vi "create systems from points.vi"(1 "points":cluster{"x":dbl, "f(x)":dbl}[](array[cluster])) -> (0 "systems of equations":T1[](array[typedef]))   [LabVIEW 2009]
uses:
  polynomial equation.ctl
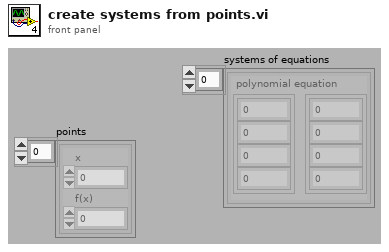
[diagram p1: front panel]
types:
  T1 = typedef "polynomial equation.ctl" = cluster{"i":dbl[], "ii":dbl[]}
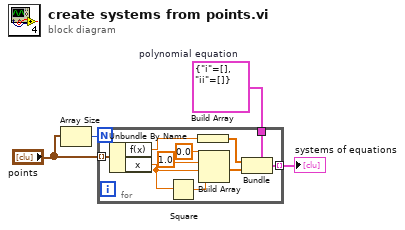
[diagram p0: block diagram]
diagram:
  w3 = T1 {"i"=[], "ii"=[]}  # polynomial equation
  n1 = Array Size(array="points") -> (size(s)=w2:i32)
  n2 = for {
    N: w2 -> [_]
    tunnel: "points" -> [w14] mode=indexing
    tunnel: w3 -> [w9]
    tunnel: [w6] -> w4 mode=indexing
    n3 = Unbundle By Name(w14) -> ("f(x)"=w10:dbl, "x"=w12:dbl)
    n4 = Square(x=w12) -> (x^2=w13:dbl)
    n5 = Build Array(w10) -> (w8:dbl[])
    n6 = Build Array(0.0 ("element"), 1.0 ("element"), w12, w13) -> (w7:dbl[])
    n7 = Bundle(cluster=w9, "i"=w8, "ii"=w7) -> (w6:T1)
  }
  "systems of equations" <- w4
